vi "Base64 Fast Decode 2012 NIVerified.vi"(8 "error in (no error)":errorcluster, 10 "string in (base64-encoded)":string) -> (0 "error out":errorcluster, 2 "string out (decoded)":string)   [LabVIEW 2021, in "LV WebSockets.lvlib"]
uses:
  LV WebSockets.lvlib
panel:
  # "Overview: This example demonstrates how to decode from Base64.\nRequirements: LabVIEW Base Development System 2012 (or compatible)\nInstructions:\n1. Enter Base64-encoded string\n2. Run the VI"
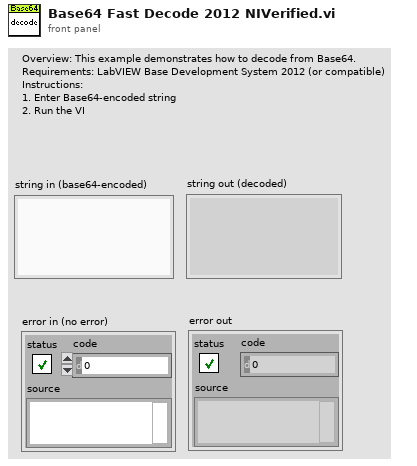
[diagram p1: front panel]
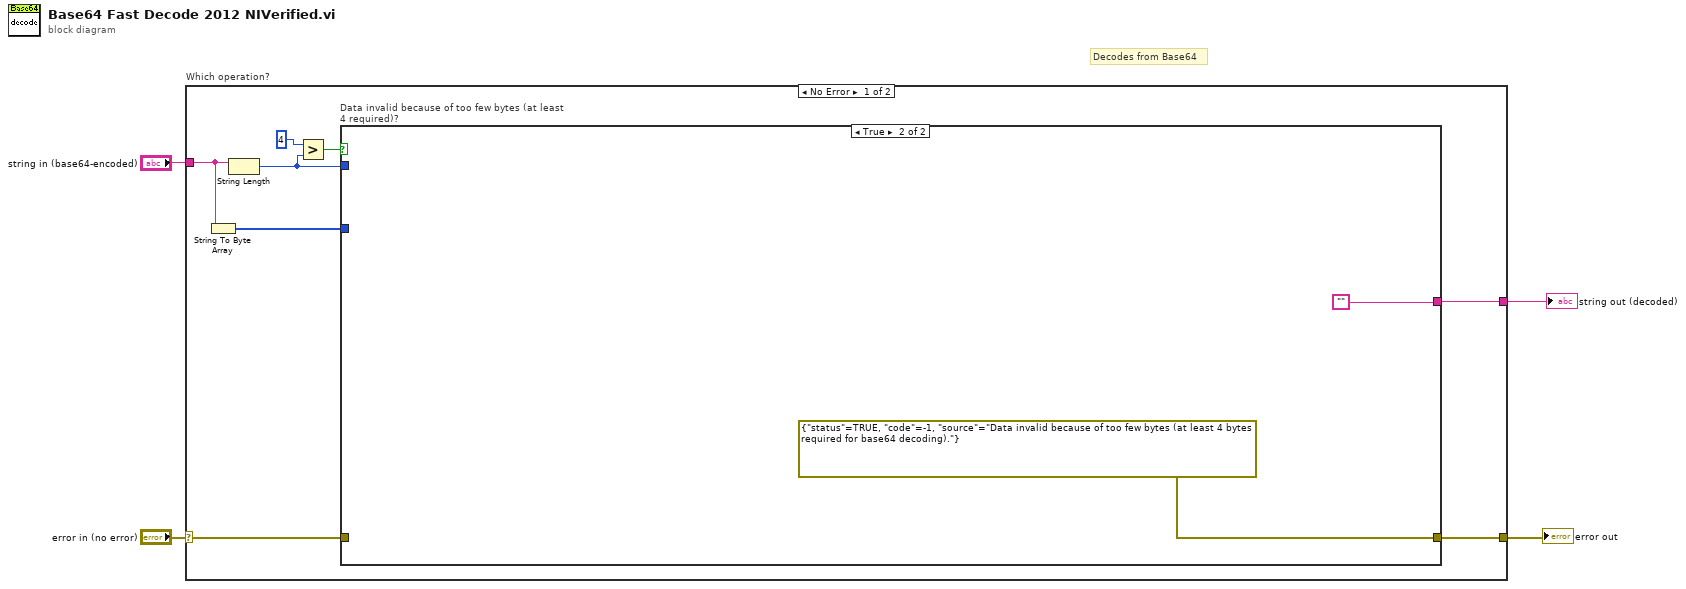
[diagram p0: block diagram]
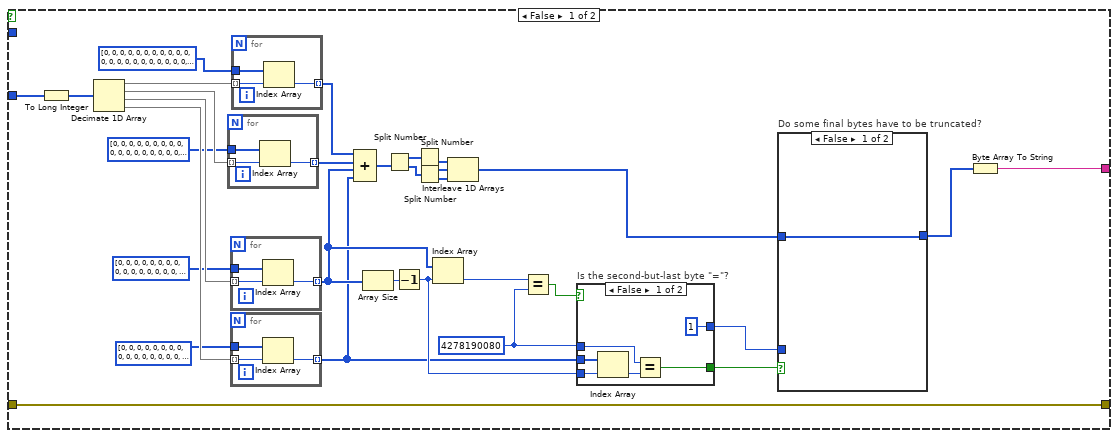
[diagram p2: hidden frame]
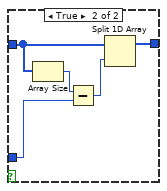
[diagram p3: hidden frame]
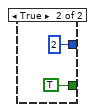
[diagram p4: hidden frame]
diagram:
  # "Decodes from Base64"
  n1 = case "Which operation?" shown="No Error" "error in (no error)" {
    selector: "error in (no error)" -> [w9 w72]
    tunnel: "string in (base64-encoded)" -> [w12 _]
    tunnel: [w8 w72] -> w3
    tunnel: [w7 _] -> w1
    frame No Error {
      n2 = String To Byte Array(string=w12) -> (unsigned byte array=w11:u8[])
      n3 = String Length(string=w12) -> (length=w6:i32)
      n4 = Greater?(x=4 ("y"), y=w6) -> (0:w10:bool)
      n5 = case "Data invalid because of too few bytes (at least 4 required)?" shown="True" w10 {
        tunnel: w11 -> [w25 _]
        tunnel: [w43 ""] -> w7
        tunnel: w6 -> [_ _]
        tunnel: [w17 errorcluster {"status"=TRUE, "code"=-1, "source"="Data invalid because of too few bytes (at least 4 bytes required for base64 decoding)."} ("error IO")] -> w8
        tunnel: w9 -> [w17 _]
        frame False {
          w18 = u32 4278190080 ("y")
          n6 = To Long Integer(number=w25) -> (32bit integer=w42:i32[])
          n7 = Decimate 1D Array(w42) -> (w31:i32[], w41:i32[], w32:i32[], w30:i32[])
          n8 = for {
            tunnel: w41 -> [w51] mode=indexing
            tunnel: u32[] [0, 0, 0, 0, 0, 0, 0, 0, 0, 0, 0, 0, 0, 0, 0, 0, 0, 0, 0, 0, 0, 0, 0, 0, 0, 0, 0, 0, 0, 0, 0, 0, 0, 0, 0, 0, 0, 0, 0, 0, 0, 0, 0, 253952, 0, 0, 0, 258048, 212992, 217088, 221184, 225280, 229376, 233472, 237568, 241664, 245760, 249856, 0, 0, 0, 0, 0, 0, 0, 0, 4096, 8192, 12288, 16384, 20480, 24576, 28672, 32768, 36864, 40960, 45056, 49152, 53248, 57344, 61440, 65536, 69632, 73728, 77824, 81920, 86016, 90112, 94208, 98304, 102400, 0, 0, 0, 0, 0, 0, 106496, 110592, 114688, 118784, 122880, 126976, 131072, 135168, 139264, 143360, 147456, 151552, 155648, 159744, 163840, 167936, 172032, 176128, 180224, 184320, 188416, 192512, 196608, 200704, 204800, 208896, 0, 0, 0, 0, 0, 0, 0, 0, 0, 0, 0, 0, 0, 0, 0, 0, 0, 0, 0, 0, 0, 0, 0, 0, 0, 0, 0, 0, 0, 0, 0, 0, 0, 0, 0, 0, 0, 0, 0, 0, 0, 0, 0, 0, 0, 0, 0, 0, 0, 0, 0, 0, 0, 0, 0, 0, 0, 0, 0, 0, 0, 0, 0, 0, 0, 0, 0, 0, 0, 0, 0, 0, 0, 0, 0, 0, 0, 0, 0, 0, 0, 0, 0, 0, 0, 0, 0, 0, 0, 0, 0, 0, 0, 0, 0, 0, 0, 0, 0, 0, 0, 0, 0, 0, 0, 0, 0, 0, 0, 0, 0, 0, 0, 0, 0, 0, 0, 0, 0, 0, 0, 0, 0, 0, 0, 0, 0, 0, 0, 0, 0, 0, 0] ("array 3") -> [w52]
            tunnel: [w50] -> w39 mode=indexing
            n9 = Index Array(array=w52, index=w51) -> (element=w50:u32)
          }
          n10 = for {
            tunnel: u32[] [0, 0, 0, 0, 0, 0, 0, 0, 0, 0, 0, 0, 0, 0, 0, 0, 0, 0, 0, 0, 0, 0, 0, 0, 0, 0, 0, 0, 0, 0, 0, 0, 0, 0, 0, 0, 0, 0, 0, 0, 0, 0, 0, 3968, 0, 0, 0, 4032, 3328, 3392, 3456, 3520, 3584, 3648, 3712, 3776, 3840, 3904, 0, 0, 0, 4278190080, 0, 0, 0, 0, 64, 128, 192, 256, 320, 384, 448, 512, 576, 640, 704, 768, 832, 896, 960, 1024, 1088, 1152, 1216, 1280, 1344, 1408, 1472, 1536, 1600, 0, 0, 0, 0, 0, 0, 1664, 1728, 1792, 1856, 1920, 1984, 2048, 2112, 2176, 2240, 2304, 2368, 2432, 2496, 2560, 2624, 2688, 2752, 2816, 2880, 2944, 3008, 3072, 3136, 3200, 3264, 0, 0, 0, 0, 0, 0, 0, 0, 0, 0, 0, 0, 0, 0, 0, 0, 0, 0, 0, 0, 0, 0, 0, 0, 0, 0, 0, 0, 0, 0, 0, 0, 0, 0, 0, 0, 0, 0, 0, 0, 0, 0, 0, 0, 0, 0, 0, 0, 0, 0, 0, 0, 0, 0, 0, 0, 0, 0, 0, 0, 0, 0, 0, 0, 0, 0, 0, 0, 0, 0, 0, 0, 0, 0, 0, 0, 0, 0, 0, 0, 0, 0, 0, 0, 0, 0, 0, 0, 0, 0, 0, 0, 0, 0, 0, 0, 0, 0, 0, 0, 0, 0, 0, 0, 0, 0, 0, 0, 0, 0, 0, 0, 0, 0, 0, 0, 0, 0, 0, 0, 0, 0, 0, 0, 0, 0, 0, 0, 0, 0, 0, 0, 0] ("array 2") -> [w69]
            tunnel: [w68] -> w23 mode=indexing
            tunnel: w32 -> [w67] mode=indexing
            n11 = Index Array(array=w69, index=w67) -> (element=w68:u32)
          }
          n12 = for {
            tunnel: u32[] [0, 0, 0, 0, 0, 0, 0, 0, 0, 0, 0, 0, 0, 0, 0, 0, 0, 0, 0, 0, 0, 0, 0, 0, 0, 0, 0, 0, 0, 0, 0, 0, 0, 0, 0, 0, 0, 0, 0, 0, 0, 0, 0, 62, 0, 0, 0, 63, 52, 53, 54, 55, 56, 57, 58, 59, 60, 61, 0, 0, 0, 4278190080, 0, 0, 0, 0, 1, 2, 3, 4, 5, 6, 7, 8, 9, 10, 11, 12, 13, 14, 15, 16, 17, 18, 19, 20, 21, 22, 23, 24, 25, 0, 0, 0, 0, 0, 0, 26, 27, 28, 29, 30, 31, 32, 33, 34, 35, 36, 37, 38, 39, 40, 41, 42, 43, 44, 45, 46, 47, 48, 49, 50, 51, 0, 0, 0, 0, 0, 0, 0, 0, 0, 0, 0, 0, 0, 0, 0, 0, 0, 0, 0, 0, 0, 0, 0, 0, 0, 0, 0, 0, 0, 0, 0, 0, 0, 0, 0, 0, 0, 0, 0, 0, 0, 0, 0, 0, 0, 0, 0, 0, 0, 0, 0, 0, 0, 0, 0, 0, 0, 0, 0, 0, 0, 0, 0, 0, 0, 0, 0, 0, 0, 0, 0, 0, 0, 0, 0, 0, 0, 0, 0, 0, 0, 0, 0, 0, 0, 0, 0, 0, 0, 0, 0, 0, 0, 0, 0, 0, 0, 0, 0, 0, 0, 0, 0, 0, 0, 0, 0, 0, 0, 0, 0, 0, 0, 0, 0, 0, 0, 0, 0, 0, 0, 0, 0, 0, 0, 0, 0, 0, 0, 0, 0, 0, 0] ("Array") -> [w66]
            tunnel: [w65] -> w21 mode=indexing
            tunnel: w30 -> [w64] mode=indexing
            n13 = Index Array(array=w66, index=w64) -> (element=w65:u32)
          }
          n14 = for {
            tunnel: w31 -> [w54] mode=indexing
            tunnel: u32[] [0, 0, 0, 0, 0, 0, 0, 0, 0, 0, 0, 0, 0, 0, 0, 0, 0, 0, 0, 0, 0, 0, 0, 0, 0, 0, 0, 0, 0, 0, 0, 0, 0, 0, 0, 0, 0, 0, 0, 0, 0, 0, 0, 16252928, 0, 0, 0, 16515072, 13631488, 13893632, 14155776, 14417920, 14680064, 14942208, 15204352, 15466496, 15728640, 15990784, 0, 0, 0, 0, 0, 0, 0, 0, 262144, 524288, 786432, 1048576, 1310720, 1572864, 1835008, 2097152, 2359296, 2621440, 2883584, 3145728, 3407872, 3670016, 3932160, 4194304, 4456448, 4718592, 4980736, 5242880, 5505024, 5767168, 6029312, 6291456, 6553600, 0, 0, 0, 0, 0, 0, 6815744, 7077888, 7340032, 7602176, 7864320, 8126464, 8388608, 8650752, 8912896, 9175040, 9437184, 9699328, 9961472, 10223616, 10485760, 10747904, 11010048, 11272192, 11534336, 11796480, 12058624, 12320768, 12582912, 12845056, 13107200, 13369344, 0, 0, 0, 0, 0, 0, 0, 0, 0, 0, 0, 0, 0, 0, 0, 0, 0, 0, 0, 0, 0, 0, 0, 0, 0, 0, 0, 0, 0, 0, 0, 0, 0, 0, 0, 0, 0, 0, 0, 0, 0, 0, 0, 0, 0, 0, 0, 0, 0, 0, 0, 0, 0, 0, 0, 0, 0, 0, 0, 0, 0, 0, 0, 0, 0, 0, 0, 0, 0, 0, 0, 0, 0, 0, 0, 0, 0, 0, 0, 0, 0, 0, 0, 0, 0, 0, 0, 0, 0, 0, 0, 0, 0, 0, 0, 0, 0, 0, 0, 0, 0, 0, 0, 0, 0, 0, 0, 0, 0, 0, 0, 0, 0, 0, 0, 0, 0, 0, 0, 0, 0, 0, 0, 0, 0, 0, 0, 0, 0, 0, 0, 0, 0] ("array 4") -> [w55]
            tunnel: [w53] -> w40 mode=indexing
            n15 = Index Array(array=w55, index=w54) -> (element=w53:u32)
          }
          n16 = Compound Arithmetic op=ADD(w40, w39, w23, w21) -> (w37:u32[])
          n17 = Array Size(array=w23) -> (size(s)=w24:i32)
          n18 = Split Number(x=w37) -> (hi(x)=w38:u16[], lo(x)=w36:u16[])
          n19 = Decrement(x=w24) -> (x-1=w22:i32)
          n20 = Split Number(x=w38) -> (lo(x)=w33:u8[])  [unwired: 1 out]
          n21 = Split Number(x=w36) -> (hi(x)=w34:u8[], lo(x)=w35:u8[])
          n22 = Index Array(array=w23, index=w22) -> (element=w20:u32)
          n23 = Interleave 1D Arrays(w33, w34, w35) -> (w16:u8[])
          n24 = Equal?(x=w20, y=w18) -> (x = y?=w19:bool)
          n25 = case "Is the second-but-last byte \"=\"?" shown="False" w19 {
            tunnel: w22 -> [w61 _]
            tunnel: w21 -> [w60 _]
            tunnel: w18 -> [w58 _]
            tunnel: [w57 TRUE] -> w15
            tunnel: [1 2] -> w14
            frame False {
              n26 = Index Array(array=w60, index=w61) -> (element=w59:u32)
              n27 = Equal?(x=w58, y=w59) -> (x = y?=w57:bool)
            }
            frame True {
            }
          }
          n28 = case "Do some final bytes have to be truncated?" shown="False" w15 {
            tunnel: w16 -> [w44 w47]
            tunnel: w14 -> [_ w49]
            tunnel: [w44 w45] -> w13
            frame False {
            }
            frame True {
              n29 = Array Size(array=w47) -> (size(s)=w48:i32)
              n30 = Subtract(x=w48, y=w49) -> (x-y=w46:i32)
              n31 = Split 1D Array(array=w47, index=w46) -> (first subarray=w45:u8[])  [unwired: 1 out]
            }
          }
          n32 = Byte Array To String(unsigned byte array=w13) -> (string=w43:string)
        }
        frame True {
        }
      }
    }
    frame Error {
    }
  }
  "error out" <- w3
  "string out (decoded)" <- w1
